vi "Read Attributes.vi"(11 "Amt_fb_user Msg":refnum<class "Amt_fb_user Msg.lvclass">) -> (2 "Payload":T1)   [LabVIEW 2025, in "Database_handler.lvlib" / "Amt_fb_user Msg.lvclass"]
uses:
  Amt_fb_user Msg.lvclass
  Amt_fb_user Msg.lvclass/Amt_fb_user Msg.ctl
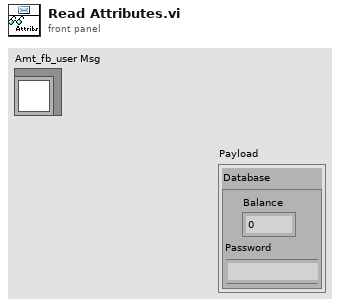
[diagram p1: front panel]
types:
  T1 = cluster{"Database":cluster{"Balance":dbl, "Password":string}}
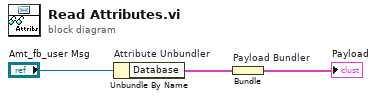
[diagram p0: block diagram]
diagram:
  n1 = Unbundle By Name "Attribute Unbundler"("Amt_fb_user Msg") -> ("Database"=w1:cluster{"Balance":dbl, "Password":string})
  n2 = Bundle "Payload Bundler"("Database"=w1) -> (→"Payload":T1)  [unwired: 1 in]
